vi "Operate Sample Process Library.vi"() -> ()   [LabVIEW 2013]
doc: "This utility VI is used to deploy and undeploy the \"sample process.lib\" in the project tree.\nYou can use this utility VI and monitor the changes in \"Simple Shared Variable and Event Monitor\" example."
uses:
  <vilib>/lvdsc/NI_DSC.lvlib
panel:
  out "Operation Log":i32(listbox)
  out "Error Out":errorcluster
  in  "Stop Button":bool
  in  "Undeploy Sample Process":bool
  in  "Deploy Sample Process":bool
  # "Sample Process.lib"
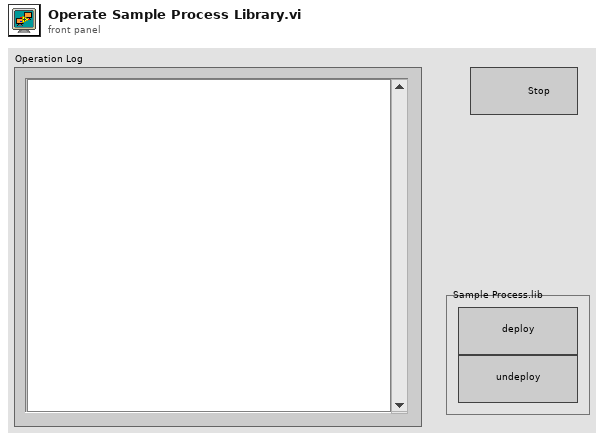
[diagram p1: front panel]
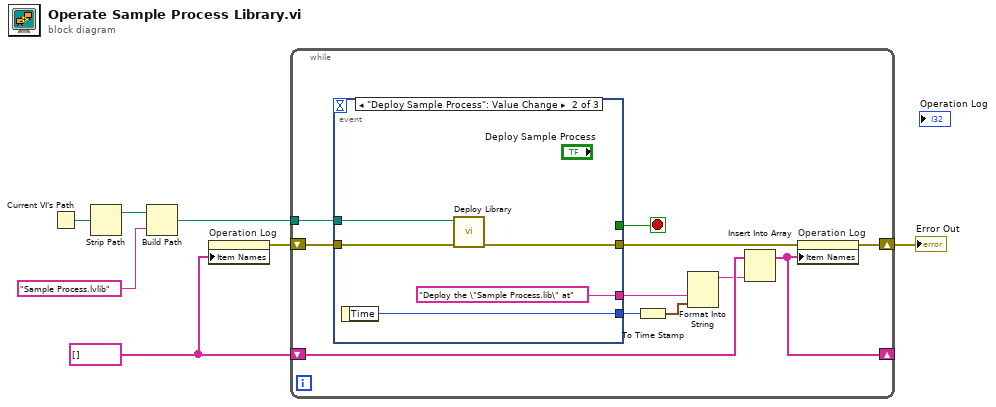
[diagram p0: block diagram]
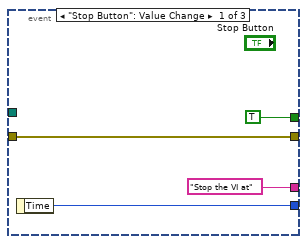
[diagram p2: hidden frame]
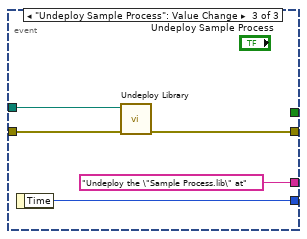
[diagram p3: hidden frame]
diagram:
  w1 = string[] [] ("Item Names")
  n1 = Current VI's Path() -> (path=w6:path)
  n2 = Strip Path(path=w6) -> (stripped path=w7:path)  [unwired: 1 out]
  n3 = Build Path(base path=w7, name or relative path="Sample Process.lvlib") -> (appended path=w5:path)
  n4 = property on="Operation Log" class="LstBox (strict)"("Item Names"=w1) -> (error out=w2:errorcluster)  [unwired: 2 in, 1 out]
  n5 = while {
    tunnel: w5 -> [w17]
    shift-right: [w14] -> w4
    shift-left: w2 -> [w16]
    shift-right: [w12] -> _
    shift-left: w1 -> [w13]
    stop <- w18 stop-if-true
    n6 = event shown="[1] \"Deploy Sample Process\": Value Change" {
      selector: _ -> [_ _ _]
      dyn-events: _ -> [_ _ _]
      timeout: _ -> [_ _ _]
      tunnel: [TRUE _ _] -> w18
      tunnel: w17 -> [_ w27 w32]
      tunnel: w16 -> [w21 w26 w30]
      tunnel: [w21 w25 w31] -> w15
      tunnel: ["Stop the VI at" ("name or relative path") "Deploy the \"Sample Process.lib\" at" ("name or relative path") "Undeploy the \"Sample Process.lib\" at" ("name or relative path")] -> w10
      tunnel: [w19 w24 w29] -> w9
      event "Stop Button": Value Change {
        n7 = event-data() -> ("Time"=w19:u32)  [unwired: 1 in]
      }
      event "Deploy Sample Process": Value Change {
        n8 = event-data() -> ("Time"=w24:u32)  [unwired: 1 in]
        n9 = call <vilib>:"Deploy Library.vi"("error in (no error)"=w26, "library path"=w27) -> ("error out"=w25:errorcluster)  [unwired: 7 in]
      }
      event "Undeploy Sample Process": Value Change {
        n10 = event-data() -> ("Time"=w29:u32)  [unwired: 1 in]
        n11 = call <vilib>:"Undeploy Library.vi"("error in (no error)"=w30, "library path"=w32) -> ("error out"=w31:errorcluster)  [unwired: 7 in]
      }
    }
    n12 = To Time Stamp(1:w9) -> (0:w11:timestamp)
    n13 = Format Into String(w10, w11) -> (resulting string=w8:string)  [unwired: 3 in, 1 out]
    n14 = Insert Into Array(array=w13, new element=w8) -> (w12:string[])  [unwired: 1 in]
    n15 = property on="Operation Log" class="LstBox (strict)"(error in=w15, "Item Names"=w12) -> (error out=w14:errorcluster)  [unwired: 1 in, 1 out]
  }
  "Error Out" <- w4
